vi "syscontrol.vi"() -> ()   [LabVIEW 2019]
uses:
  <vilib>/Platform/TimedLoop/XDataNode/timing_clust.ctl
  <vilib>/Platform/TimedLoop/XDataNode/nitl_modes.ctl
  <vilib>/Platform/TimedLoop/XDataNode/wakeup.ctl
  <vilib>/Platform/TimedLoop/XDataNode/XDataNode.xnode
  <vilib>/Platform/TimedLoop/XDataNode/XDNodeRunTimeDep.lvlib
panel:
  in  "prefiltro":bool
  out "graph signals":dynamicdata(graph)
  in  "reference":dbl
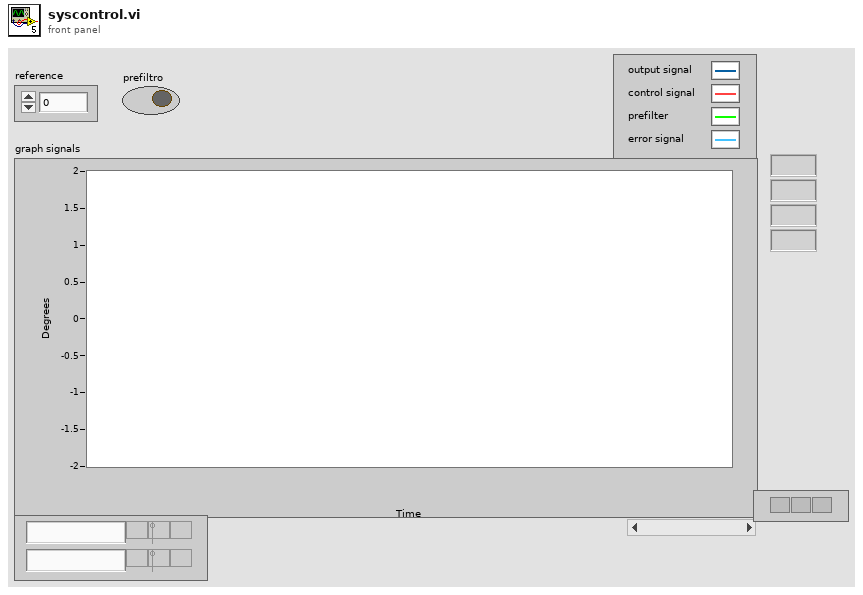
[diagram p1: front panel]
types:
  T1 = typedef "XDNodeRunTimeDep.lvlib/timing_clust.ctl" = cluster{"Expected End [f-1]":u64, "Actual End [f-1]":u64, "Finished Late? [f-1]":bool, "Expected End [i-1]":u64, "Actual End [i-1]":u64, "Finished Late? [i-1]":bool, "Expected Start [i]":u64, "Actual Start [i]":u64, "Expected Start [f]":u64, "Actual Start [f]":u64, "Source Name":string, "Structure Name":string, "Period":i64, "Deadline":i64, "Offset":i64, "Start":i64, "Priority":i32, "Timeout":i32, "Mode":T2, "Wakeup Reason":T3, "Error":errorcluster, "Source Type":string, "Secondary Source Type":string, "Global End Time":u64, "Global Start Time":u64, "Frame Duration":u64, "Iteration Duration":u64, "Assigned CPU":i32, "I/O Scan Engine Mode":u32}
  T2 = typedef "XDNodeRunTimeDep.lvlib/nitl_modes.ctl" = enum32{"No Change", "Process missed periods, maintain original phase", "Discard missed periods, maintain original phase", "Process missed periods, ignore original phase", "Discard missed periods, ignore original phase"}
  T3 = typedef "XDNodeRunTimeDep.lvlib/wakeup.ctl" = enum32{"Normal", "Aborted", "Asynchronous wakeup", "Timing source error", "Timed loop error", "Timeout"}
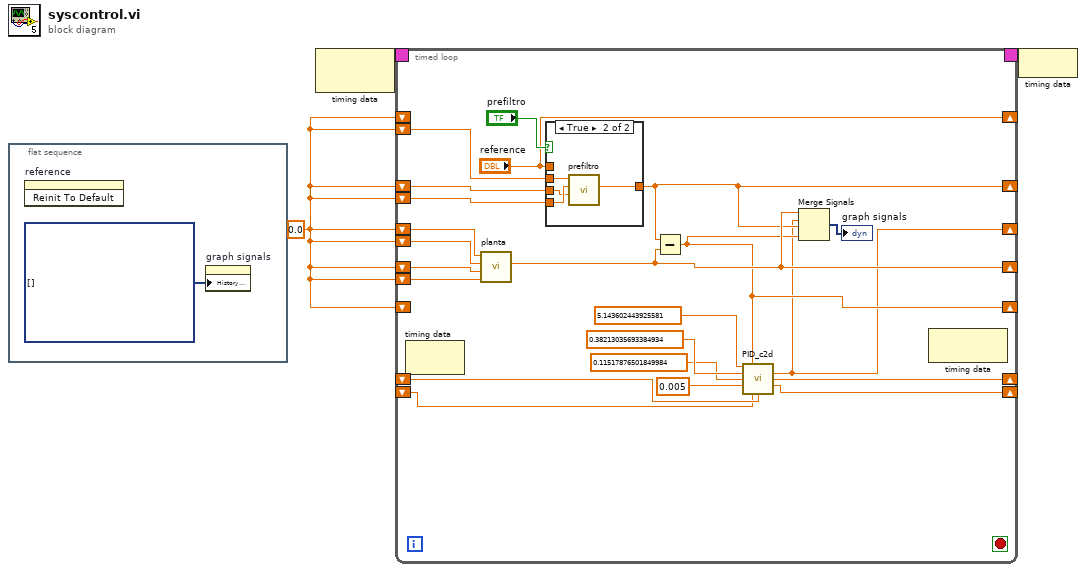
[diagram p0: block diagram]
diagram:
  w1 = 0.0 ("Referencia")
  n1 = flat-sequence {
    frame #0 {
      n2 = invoke on="reference" class="DigNum (strict)" method="Reinit To Default"() -> ()  [unwired: 3 in, 3 out]
      n3 = property on="graph signals" class="WFChart (strict)"("History Data"=dynamicdata[] []) -> ()  [unwired: 2 in, 2 out]
    }
  }
  n4 = node-c288() -> (w3:T1)  [unwired: 1 in]
  n5 = timed-loop {
    timing: w3 -> [_]
    timing-out: [_] -> w2
    shift-right: [w17] -> _
    shift-left: w1 -> [w18]
    shift-right: [w5] -> _
    shift-left: w1 -> [w15]
    shift-right: [w22] -> _
    shift-left: w1 -> [w25]
    shift-right: ["reference"] -> _
    shift-left: w1 -> [_]
    shift-left: w1 -> [w20]
    shift-left: w1 -> [w19]
    shift-left: w1 -> [w26]
    shift-left: w1 -> [w24]
    shift-right: [w9] -> _
    shift-left: w1 -> [_]
    shift-right: [w13] -> _
    shift-left: _ -> [w12]
    shift-right: [w11] -> _
    shift-left: _ -> [w10]
    stop <- _ stop-if-true
    n6 = node-c288() -> ()  [unwired: 1 in, 1 out]
    n7 = call "planta.vi"("yk-2"=w24, "yk-1"=w25, "mk-2"=w26, "mk-1"=w15) -> ("yk"=w22:dbl)  [unwired: 7 in]
    n8 = case shown="True" "prefiltro" {
      tunnel: w20 -> [_ w31]
      tunnel: w19 -> [_ w30]
      tunnel: w18 -> [_ w29]
      tunnel: [w27 w28] -> w17
      tunnel: "reference" -> [w27 _]
      frame False {
      }
      frame True {
        n9 = call "prefiltro.vi"("pk-1"=w29, "pk-2"=w30, "rk-2"=w31) -> ("pk"=w28:dbl)  [unwired: 8 in]
      }
    }
    n10 = Subtract(x=w17, y=w22) -> (x-y=w9:dbl)
    n11 = call "PID_c2d.vi"("kp"=5.143602443925581, "ek"=w9, "ti"=0.38213035693384934 ("kp"), "td"=0.11517876501849984 ("kp"), "Ts"=0.005 ("kp"), "u2k-1"=w10, "u1k-1"=w12) -> ("uk"=w5:dbl, "u1k"=w13:dbl, "u2k"=w11:dbl)  [unwired: 6 in]
    n12 = Merge Signals(w22, w5, w17, w9) -> (→"graph signals":dynamicdata)
    n13 = node-c288() -> ()  [unwired: 1 in, 1 out]
  }
  n14 = node-c288(w2) -> ()
